vi "Contour Line_Main (Scalar).vi"(8 "height":dbl, 9 "Z":dbl[][](array[numeric]), 10 "Y":dbl[][](array[numeric]), 11 "X":dbl[][](array[numeric])) -> (2 "Contour Line":T1, 3 "Contour Graph":cluster{dbl[], dbl[]}(graph))   [LabVIEW 2017, in "NI_AAL_Geometry.lvlib"]
uses:
  <vilib>/Analysis/NI_AAL_Geometry.lvlib
  <vilib>/Analysis/geometry.llb/Contour Lines Control.ctl
  <vilib>/Analysis/geometry.llb/Contour Line Segment.ctl
panel:
  # "Contour Line"
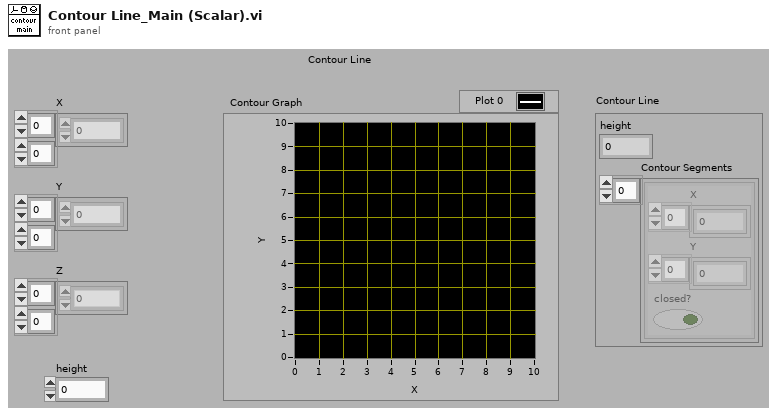
[diagram p1: front panel]
types:
  T1 = typedef "NI_AAL_Geometry.lvlib/Contour Lines Control.ctl" = cluster{"height":dbl, "Contour Segments":T2[]}
  T2 = typedef "NI_AAL_Geometry.lvlib/Contour Line Segment.ctl" = cluster{"X":dbl[], "Y":dbl[], "closed?":bool}
  T3 = cluster{"index 1":cluster{"row":i32, "column":i32}, "index 2":cluster{"row":i32, "column":i32}}[]
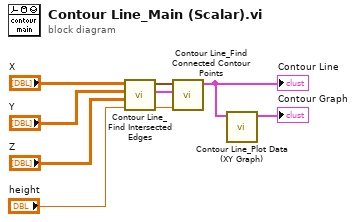
[diagram p0: block diagram]
diagram:
  n1 = call <vilib>:"Contour Line_Find Intersected Edges.vi"("height in"="height", "Z"="Z", "Y"="Y", "X"="X") -> ("height out"=w7:dbl, "Intersected Edges"=w8:T3, "Contour Points"=w9:cluster{"x":dbl, "y":dbl}[])  [unwired: 5 out]
  n2 = call <vilib>:"Contour Line_Find Connected Contour Points.vi"("height"=w7, "Intersected Edges"=w8, "Contour Points"=w9) -> ("Contour Line"=w1:T1)  [unwired: 8 out]
  "Contour Line" <- w1
  n3 = call <vilib>:"Contour Line_Plot Data (XY Graph).vi"("Contour Line"=w1) -> ("Contour Graph"=→"Contour Graph":cluster{dbl[], dbl[]})  [unwired: 10 in]
